vi "PXF4_get_cont_mode.vi"(8 "error in":errorcluster, 11 "Modbus Master in":refnum<class "Modbus Master.lvclass">) -> (0 "error out":errorcluster, 2 "mode":enum16{"Auto", "Manual"}(ring), 3 "Modbus Master out":refnum<class "Modbus Master.lvclass">)   [LabVIEW 2019]
uses:
  <vilib>/NI/Modbus Library/API/Master/Modbus Master.lvclass
panel:
  out "raw":u16
  out "register values":u16[](array[numeric])
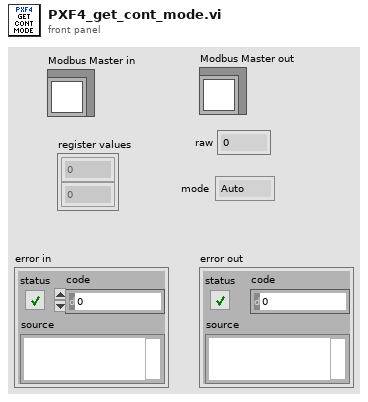
[diagram p1: front panel]
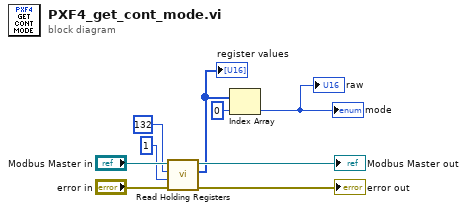
[diagram p0: block diagram]
diagram:
  n1 = call-dynamic "Read Holding Registers.vi"("error in"="error in", "number of inputs"=u16 1, "starting address"=u16 132, "Modbus master in"="Modbus Master in") -> ("error out"=→"error out":errorcluster, "register values"=w1:u16[], "Modbus master out"=→"Modbus Master out":refnum<class "Modbus Master.lvclass">)  [unwired: 5 in]
  "register values" <- w1
  n2 = Index Array(array=w1, index=0) -> (element=→"raw" →"mode":u16)
